vi "split3.vi"(7 "Array of Waveform In":waveform(i16)[](array[waveform])) -> (1 "Sync":waveform(i16), 3 "Array of Waveform":waveform(i16)[](array[waveform]))   [LabVIEW 2010]
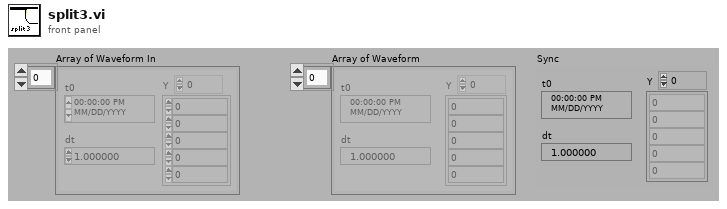
[diagram p1: front panel]
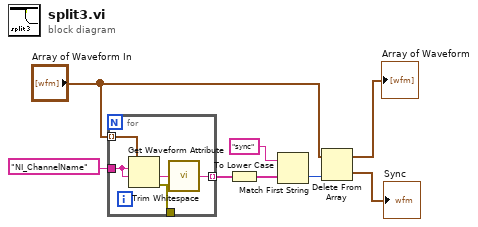
[diagram p0: block diagram]
diagram:
  n1 = for {
    tunnel: "Array of Waveform In" -> [w13] mode=indexing
    tunnel: "NI_ChannelName" ("name") -> [w11]
    tunnel: [w10] -> w2 mode=indexing
    tunnel: [w9] -> _
    n2 = Get Waveform Attribute(5:w11, 6:w11, 7:w13) -> (0:w9:errorcluster, 1:w12:string)  [unwired: 1 in, 2 out]
    n3 = call <vilib>:"Trim Whitespace.vi"("string"=w12) -> ("trimmed string"=w10:string)  [unwired: 1 in]
  }
  n4 = To Lower Case(string=w2) -> (all lower case string=w7:string[])
  n5 = Match First String(2:w7, 3:"sync" ("name")) -> (0:w4:i32)  [unwired: 1 out]
  n6 = Delete From Array(array="Array of Waveform In", index=w4) -> (deleted portion=→"Sync":waveform(i16), array with subset deleted=→"Array of Waveform":waveform(i16)[])  [unwired: 1 in]
